vi "בדיקת מפל מתח בין הדקי הממסר תחת עומס 6.vi"(8 "error":errorcluster, 11 "Path for Log":path) -> (0 "error IO":errorcluster, 1 "בטווח כן/לא":bool, 2 "מפל מתח בין דקי הממסר תחת עומס":dbl, 3 "תוצאה זמנית":dbl)   [LabVIEW 2014]
uses:
  M9700 Driver/85/vi.lib/M9700 Modbus.llb/CTL Register Address.ctl
  M9700 Driver/86/vi.lib/M9700 Modbus.llb/CTL CMD Register.ctl
  <vilib>/Instr/_visa.llb/VISA Configure Serial Port (Instr).vi
  <vilib>/DAQmx/create/channels.llb/DAQmx Create Channel (DO-Digital Output).vi
  <vilib>/DAQmx/write.llb/DAQmx Write (Digital Bool 1Line 1Point).vi
panel:
  out "progress":dbl(slide) min=0.0 max=10.0 scale=0.0..10.0
  in  "stop":bool
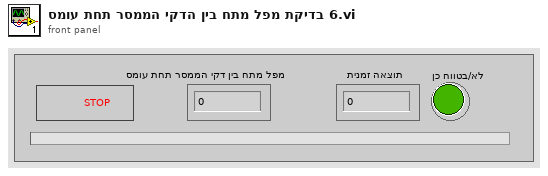
[diagram p1: front panel]
types:
  T1 = enum32{"Invalid", "Standard", "Closed", "Hidden", "Minimized", "Maximized"}
  T2 = typedef "CTL CMD Register.ctl" = u8
  T3 = typedef "CTL Register Address.ctl" = u16
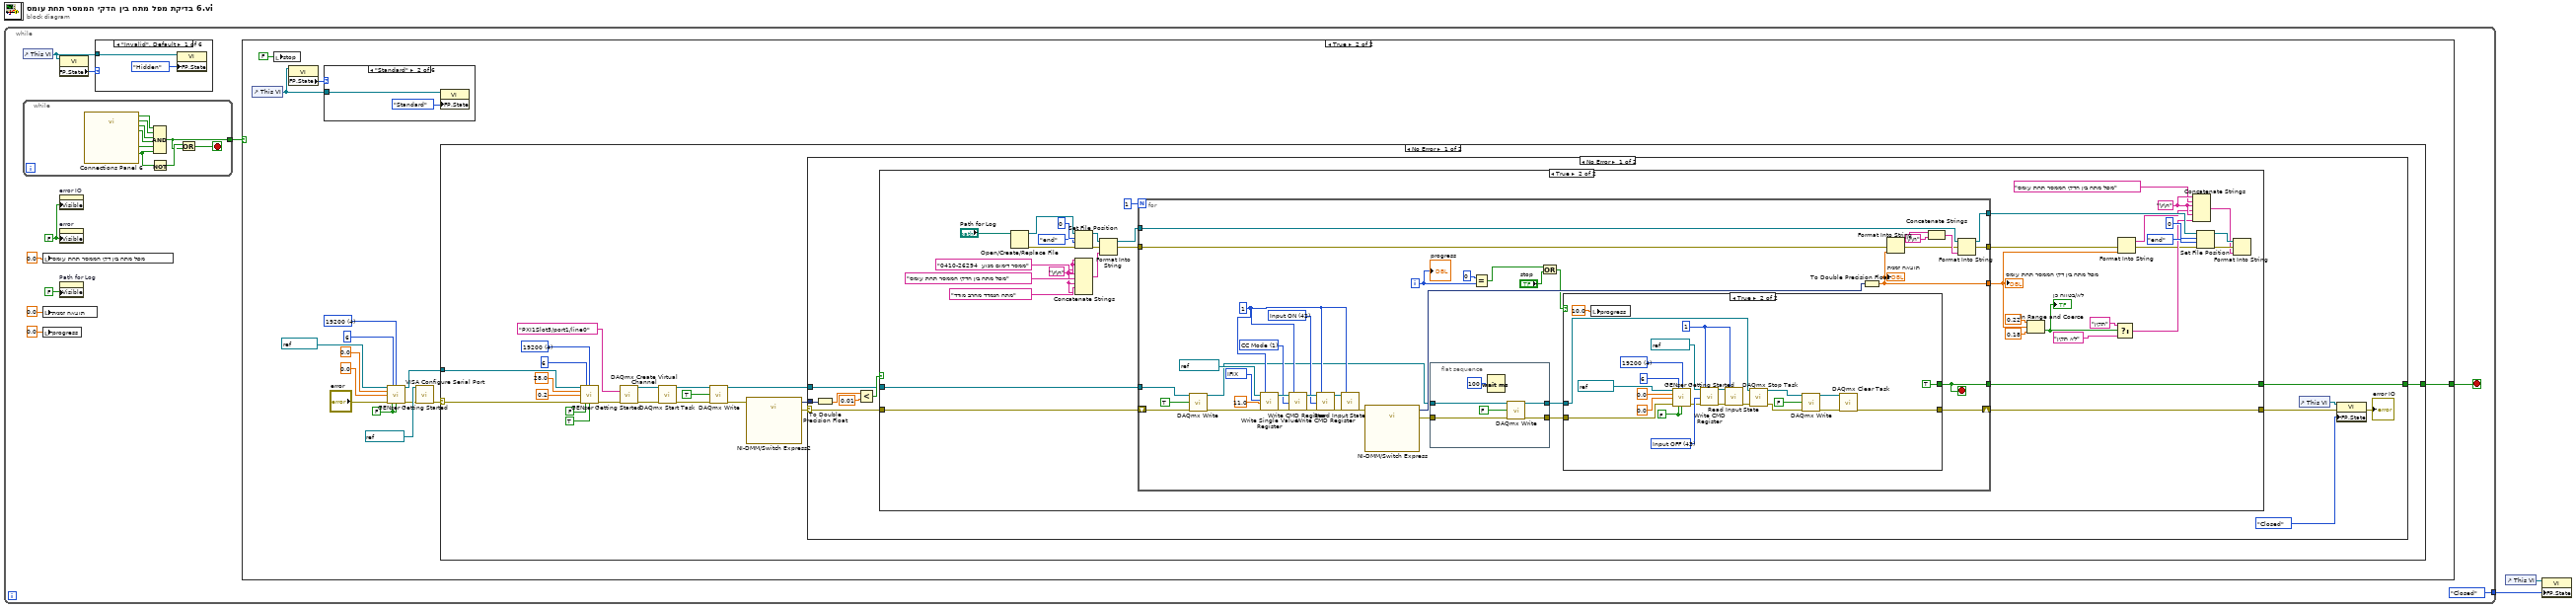
[diagram p0: block diagram]
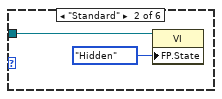
[diagram p2: hidden frame]
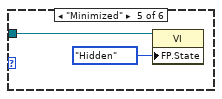
[diagram p5: hidden frame]
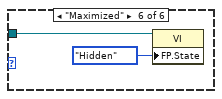
[diagram p6: hidden frame]
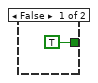
[diagram p7: hidden frame]
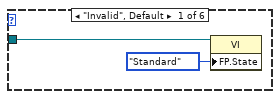
[diagram p8: hidden frame]
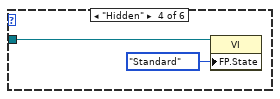
[diagram p10: hidden frame]
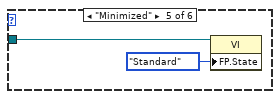
[diagram p11: hidden frame]
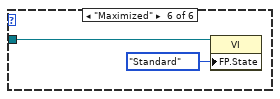
[diagram p12: hidden frame]
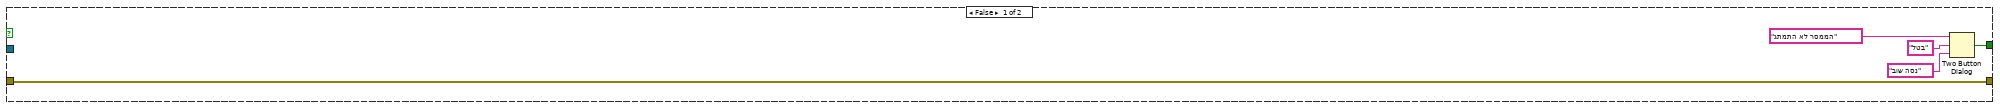
[diagram p13: hidden frame]
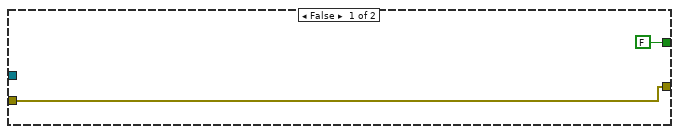
[diagram p14: hidden frame]
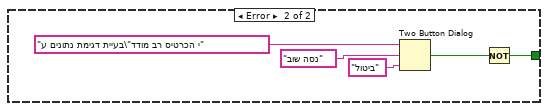
[diagram p15: hidden frame]
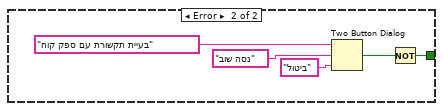
[diagram p16: hidden frame]
diagram:
  n1 = while {
    tunnel: [T1."Closed" ("Front Panel Window:State")] -> w1
    stop <- w12 stop-if-true
    w8 = FALSE ("Visible")
    n2 = control-ref of="This VI"() -> (w5:refnum<vi>)
    n3 = while {
      tunnel: [w13] -> w6
      stop <- w15 stop-if-true
      n4 = call "Connections Panel 6.vi"() -> ("Input Name 10"=w17:bool, "Input Name 6"=w21:bool, "Input Name 7"=w20:bool, "Input Name 8"=w19:bool, "Input Name 9"=w18:bool, "OK"=w14:bool)  [unwired: 13 in, 1 out]
      n5 = Not(x=w14) -> (.not. x?=w16:bool)
      n6 = Compound Arithmetic op=AND(w21, w20, w19, w18, w17, w14) -> (w13:bool)
      n7 = Or(x=w16, y=w13) -> (x .or. y?=w15:bool)
    }
    n8 = local write "מפל מתח בין דקי הממסר תחת עומס"(0.0 ("מפל מתח בין דקי הממסר תחת עומס")) -> ()
    n9 = local write "תוצאה זמנית"(0.0 ("תוצאה זמנית")) -> ()
    n10 = local write "progress"(0.0 ("progress")) -> ()
    n11 = property class="VI"(reference=w5) -> ("FP.State"=w4:T1)  [unwired: 1 in, 2 out]
    n12 = property on="error IO" class="Clust (strict)"("Visible"=w8) -> ()  [unwired: 2 in, 2 out]
    n13 = property on="error" class="Clust (strict)"("Visible"=w8) -> ()  [unwired: 2 in, 2 out]
    n14 = property on="Path for Log" class="Path"("Visible"=FALSE) -> ()  [unwired: 2 in, 2 out]
    n15 = case shown="\"Invalid\", Default" w4 {
      tunnel: w5 -> [w22 w24 _ _ w26 w28]
      frame "Invalid", Default {
        n16 = property class="VI"(reference=w22, "FP.State"=T1."Hidden" ("Front Panel Window:State")) -> ()  [unwired: 1 in, 2 out]
      }
      frame "Standard" {
        n17 = property class="VI"(reference=w24, "FP.State"=T1."Hidden" ("Front Panel Window:State")) -> ()  [unwired: 1 in, 2 out]
      }
      frame "Closed" {
      }
      frame "Hidden" {
      }
      frame "Minimized" {
        n18 = property class="VI"(reference=w26, "FP.State"=T1."Hidden" ("Front Panel Window:State")) -> ()  [unwired: 1 in, 2 out]
      }
      frame "Maximized" {
        n19 = property class="VI"(reference=w28, "FP.State"=T1."Hidden" ("Front Panel Window:State")) -> ()  [unwired: 1 in, 2 out]
      }
    }
    n20 = case shown="True" w6 {
      tunnel: [TRUE w38] -> w12
      frame False {
      }
      frame True {
        w35 = FALSE ("Output On (T)")
        w42 = u16 4 items=["1200", "2400", "4800", "9600", "19200"] ("BAUD")
        n21 = control-ref of="This VI"() -> (w31:refnum<vi>)
        n22 = local write "stop"(FALSE ("stop")) -> ()
        n23 = property class="VI"(reference=w31) -> ("FP.State"=w32:T1)  [unwired: 1 in, 2 out]
        n24 = case shown="\"Standard\"" w32 {
          tunnel: w31 -> [w46 w48 _ w50 w52 w54]
          frame "Invalid", Default {
            n25 = property class="VI"(reference=w46, "FP.State"=T1."Standard" ("Front Panel Window:State")) -> ()  [unwired: 1 in, 2 out]
          }
          frame "Standard" {
            n26 = property class="VI"(reference=w48, "FP.State"=T1."Standard" ("Front Panel Window:State")) -> ()  [unwired: 1 in, 2 out]
          }
          frame "Closed" {
          }
          frame "Hidden" {
            n27 = property class="VI"(reference=w50, "FP.State"=T1."Standard" ("Front Panel Window:State")) -> ()  [unwired: 1 in, 2 out]
          }
          frame "Minimized" {
            n28 = property class="VI"(reference=w52, "FP.State"=T1."Standard" ("Front Panel Window:State")) -> ()  [unwired: 1 in, 2 out]
          }
          frame "Maximized" {
            n29 = property class="VI"(reference=w54, "FP.State"=T1."Standard" ("Front Panel Window:State")) -> ()  [unwired: 1 in, 2 out]
          }
        }
        n30 = call "GENser Getting Started.vi"("VISA"=refnum<visa-resource-name> "COM6", "GEN Addr"=i16 6, "BAUD"=w42, "Voltage Limit"=0.0, "Current Limit"=0.0, "error"="error", "Reset (T)"=w35, "Output On (T)"=w35) -> ("VISA out"=w44:refnum<visa-resource-name>, "error out"=w33:errorcluster)  [unwired: 4 in, 2 out]
        n31 = call-poly "VISA Configure Serial Port"("VISA resource name"=refnum<visa-resource-name> "COM13", "error in (no error)"=w33) -> ("error out"=w36:errorcluster)  [unwired: 4 in, 9 out]
        n32 = case shown="No Error" w36 {
          selector: w36 -> [w72 _]
          tunnel: w44 -> [w75 _]
          tunnel: [w74 w203] -> w38
          frame No Error {
            w66 = u16 4 items=["1200", "2400", "4800", "9600", "19200"] ("BAUD")
            n33 = call "GENser Getting Started.vi"("VISA"=w75, "GEN Addr"=i16 6, "BAUD"=w66, "Voltage Limit"=28.0, "Current Limit"=0.2, "error"=w72, "Reset (T)"=FALSE, "Output On (T)"=TRUE) -> ("error out"=w61:errorcluster)  [unwired: 4 in, 3 out]
            n34 = call-poly <vilib>:"DAQmx Create Virtual Channel.vi"("lines"=tag "PXI1Slot5/port1/line0", "error in"=w61) -> ("task out"=w64:refnum<k21>, "error out"=w65:errorcluster)  [unwired: 12 in]
            n35 = call <vilib>:"DAQmx Start Task.vi"("task/channels in"=w64, "error in"=w65) -> ("task out"=w60:refnum<k21>, "error out"=w58:errorcluster)  [unwired: 12 in]
            n36 = call-poly <vilib>:"DAQmx Write.vi"("task/channels in"=w60, "data"=TRUE, "error in"=w58) -> ("task out"=w59:refnum<k21>, "error out"=w57:errorcluster)  [unwired: 10 in, 1 out]
            n37 = call "NI-DMM/Switch Express2"("error in"=w57) -> ("signals out"=w73:dynamicdata, "error out"=w62:errorcluster)  [unwired: 16 in, 1 out]
            n38 = case shown="No Error" w62 {
              selector: w62 -> [w84 _]
              tunnel: [w83 w198] -> w74
              tunnel: w73 -> [w86 _]
              tunnel: w59 -> [w77 _]
              frame No Error {
                n39 = To Double Precision Float(number=w86) -> (double precision float=w82:dbl)
                n40 = Less?(x=w82, y=0.01) -> (x < y?=w85:bool)
                n41 = case shown="True" w85 {
                  tunnel: w84 -> [w91 w126]
                  tunnel: [w87 w127] -> w83
                  tunnel: [w91 w122] -> w78
                  tunnel: w77 -> [_ w123]
                  frame False {
                    n42 = Two Button Dialog(message="הממסר לא התמתג", 1:"נסה שוב" ("F button name (\"Cancel\")"), 2:"בטל" ("T button name (\"OK\")")) -> (T button?=w87:bool)
                  }
                  frame True {
                    w108 = "\r\n"
                    w111 = "\r\n"
                    n43 = Open/Create/Replace File(file path (use dialog)="Path for Log") -> (refnum out=w119:refnum<file>, error out=w118:errorcluster)  [unwired: 5 in, 1 out]
                    n44 = Set File Position(offset (in bytes) (0)=i64 0, refnum=w119, from (0:start)=enum16{"start", "end", "current"}."end", error in=w118) -> (refnum out=w115:refnum<file>, error out=w112:errorcluster)
                    n45 = Concatenate Strings(w111, w111, "0410-26294  ממסר דימום מנוע", w111, "מפל מתח בין הדקי הממסר תחת עומס", w111, "מתח הנמדד מהרב מודד", w111) -> (w117:string)
                    n46 = Format Into String(initial string=w115, error in=w112, w117) -> (resulting string=w109:refnum<file>, error out=w110:errorcluster)  [unwired: 1 in]
                    n47 = for {
                      N: 1 -> [_]
                      tunnel: [w149] -> w127
                      shift-right: [w147] -> w122
                      shift-left: w126 -> [w142]
                      tunnel: w123 -> [w143]
                      tunnel: w110 -> [w133]
                      tunnel: w109 -> [w135]
                      tunnel: [w132] -> w102
                      tunnel: [w131] -> w94
                      tunnel: [w129] -> w92
                      i -> [w146]
                      stop <- w149 stop-if-true
                      w157 = T2 42 items=["CC Mode"=1, "CV Mode"=2, "CW Mode"=3, "CR Mode"=4, "Short Mode"=26, "Set SysPara"=41, "Input ON"=42, "Input OFF"=43] ("CMD Register Value")
                      w160 = u8 1 ("Load Address")
                      w163 = T2 1 items=["CC Mode"=1, "CV Mode"=2, "CW Mode"=3, "CR Mode"=4, "Short Mode"=26, "Set SysPara"=41, "Input ON"=42, "Input OFF"=43] ("CMD Register Value")
                      w166 = T3 2561 items=["REMOTE"=1283, "ISTATE"=1296, "CMD"=2560, "IFIX"=2561, "UFIX"=2563, "PFIX"=2565, "RFIX"=2567, "IMAX"=2612, "UMAX"=2614, "PMAX"=2616, "U"=2816, "I"=2818, "MODEL"=2822, "EDITION"=2823] ("Register Address")
                      n48 = call-poly <vilib>:"DAQmx Write.vi"("task/channels in"=w143, "data"=TRUE, "error in"=w142) -> ("task out"=w141:refnum<k21>, "error out"=w130:errorcluster)  [unwired: 10 in, 1 out]
                      n49 = call "Write Single Value Register.vi"("VISA resource name"=refnum<visa-resource-name> "COM13", "Starting Address(HEX)"=w166, "Register Single Value"=sgl 11.0, "error in"=w130, "Load Address"=w160) -> ("VISA resource name out"=w165:refnum<visa-resource-name>, "error out"=w164:errorcluster)  [unwired: 13 out]
                      n50 = call "Write CMD Register.vi"("VISA resource name"=w165, "CMD Value"=w163, "error in"=w164, "Load Address"=w160) -> ("VISA resource name out"=w161:refnum<visa-resource-name>, "error out"=w158:errorcluster)  [unwired: 14 out]
                      n51 = call "Write CMD Register.vi"("VISA resource name"=w161, "CMD Value"=w157, "error in"=w158, "Load Address"=w160) -> ("VISA resource name out"=w159:refnum<visa-resource-name>, "error out"=w156:errorcluster)  [unwired: 14 out]
                      n52 = call "Read Input State.vi"("VISA resource name"=w159, "error in"=w156, "Load Address"=w160) -> ("error out"=w155:errorcluster)  [unwired: 16 out]
                      n53 = call "NI-DMM/Switch Express"("error in"=w155) -> ("signals out"=w154:dynamicdata, "error out"=w144:errorcluster)  [unwired: 16 in, 1 out]
                      n54 = flat-sequence {
                        tunnel: [w172] -> w145
                        tunnel: w144 -> [w171]
                        tunnel: w141 -> [w169]
                        tunnel: [w168] -> w139
                        frame #0 {
                          n55 = Wait (ms)(milliseconds to wait=u32 100) -> ()  [unwired: 1 out]
                          n56 = call-poly <vilib>:"DAQmx Write.vi"("task/channels in"=w169, "data"=FALSE, "error in"=w171) -> ("task out"=w168:refnum<k21>, "error out"=w172:errorcluster)  [unwired: 10 in, 1 out]
                        }
                      }
                      n57 = Equal?(x=0, y=w146) -> (x = y?=w151:bool)
                      n58 = Or(x=w151, y="stop") -> (x .or. y?=w152:bool)
                      n59 = case shown="True" w152 {
                        tunnel: [FALSE TRUE] -> w149
                        tunnel: w145 -> [w173 w191]
                        tunnel: [w173 w177] -> w147
                        tunnel: w139 -> [_ w176]
                        frame False {
                        }
                        frame True {
                          w185 = u8 1 ("Load Address")
                          w188 = T2 43 items=["CC Mode"=1, "CV Mode"=2, "CW Mode"=3, "CR Mode"=4, "Short Mode"=26, "Set SysPara"=41, "Input ON"=42, "Input OFF"=43] ("CMD Register Value")
                          w190 = FALSE ("Reset (T)")
                          w193 = u16 4 items=["1200", "2400", "4800", "9600", "19200"] ("BAUD")
                          n60 = local write "progress"(10.0 ("progress")) -> ()
                          n61 = call "GENser Getting Started.vi"("VISA"=refnum<visa-resource-name> "COM6", "GEN Addr"=i16 6, "BAUD"=w193, "Voltage Limit"=0.0, "Current Limit"=0.0, "error"=w191, "Reset (T)"=w190, "Output On (T)"=w190) -> ("error out"=w175:errorcluster)  [unwired: 4 in, 3 out]
                          n62 = call "Write CMD Register.vi"("VISA resource name"=refnum<visa-resource-name> "COM13", "CMD Value"=w188, "error in"=w175, "Load Address"=w185) -> ("VISA resource name out"=w186:refnum<visa-resource-name>, "error out"=w189:errorcluster)  [unwired: 14 out]
                          n63 = call "Read Input State.vi"("VISA resource name"=w186, "error in"=w189, "Load Address"=w185) -> ("error out"=w178:errorcluster)  [unwired: 16 out]
                          n64 = call <vilib>:"DAQmx Stop Task.vi"("task/channels in"=w176, "error in"=w178) -> ("task out"=w183:refnum<k21>, "error out"=w181:errorcluster)  [unwired: 12 in]
                          n65 = call-poly <vilib>:"DAQmx Write.vi"("task/channels in"=w183, "data"=FALSE, "error in"=w181) -> ("task out"=w180:refnum<k21>, "error out"=w179:errorcluster)  [unwired: 10 in, 1 out]
                          n66 = call <vilib>:"DAQmx Clear Task.vi"("task in"=w180, "error in"=w179) -> ("error out"=w177:errorcluster)  [unwired: 13 in]
                        }
                      }
                      n67 = To Double Precision Float(number=w154) -> (double precision float=w129:dbl)
                      "תוצאה זמנית" <- w129
                      n68 = Format Into String(error in=w133, w129) -> (resulting string=w137:string, error out=w134:errorcluster)  [unwired: 2 in]
                      n69 = Concatenate Strings(w137, "\r\n") -> (w136:string)
                      n70 = Format Into String(initial string=w135, error in=w134, w136) -> (resulting string=w132:refnum<file>, error out=w131:errorcluster)  [unwired: 1 in]
                      "progress" <- w146
                    }
                    "מפל מתח בין דקי הממסר תחת עומס" <- w92
                    n71 = In Range and Coerce(upper limit=0.22, x=w92, lower limit=0.18) -> (In Range?=w97:bool)  [unwired: 1 out]
                    "בטווח כן/לא" <- w97
                    n72 = Select(t="תקין", s=w97, f="לא תקין") -> (s? t:f=w96:string)
                    n73 = Format Into String(error in=w94, w92) -> (resulting string=w101:string, error out=w95:errorcluster)  [unwired: 2 in]
                    n74 = Concatenate Strings(w108, "מפל מתח בין הדקי הממסר תחת עומס" ("string"), w108, w101, w108, w96) -> (w103:string)
                    n75 = Set File Position(offset (in bytes) (0)=i64 0, refnum=w102, from (0:start)=enum16{"start", "end", "current"}."end", error in=w95) -> (refnum out=w105:refnum<file>, error out=w104:errorcluster)
                    n76 = Format Into String(initial string=w105, error in=w104, w103) -> ()  [unwired: 1 in, 2 out]
                  }
                }
                n77 = control-ref of="This VI"() -> (w80:refnum<vi>)
                n78 = property class="VI"(reference=w80, error in=w78, "FP.State"=T1."Closed" ("Front Panel Window:State")) -> (error out=→"error IO":errorcluster)  [unwired: 1 out]
              }
              frame Error {
                n79 = Two Button Dialog(message="בעיית דגימת נתונים ע\"י הכרטיס רב מודד", 1:"ביטול" ("F button name (\"Cancel\")"), 2:"נסה שוב" ("T button name (\"OK\")")) -> (T button?=w199:bool)
                n80 = Not(x=w199) -> (.not. x?=w198:bool)
              }
            }
          }
          frame Error {
            n81 = Two Button Dialog(message="בעיית תקשורת עם ספק קוח", 1:"ביטול" ("F button name (\"Cancel\")"), 2:"נסה שוב" ("T button name (\"OK\")")) -> (T button?=w204:bool)
            n82 = Not(x=w204) -> (.not. x?=w203:bool)
          }
        }
      }
    }
  }
  n83 = control-ref of="This VI"() -> (w2:refnum<vi>)
  n84 = property class="VI"(reference=w2, "FP.State"=w1) -> ()  [unwired: 1 in, 2 out]
